vi "FPGA-MAIN.vi"() -> ()   [LabVIEW 2013]
uses:
  <vilib>/LabVIEW Targets/FPGA/cRIO/shared/nicrio_ModuleControls/nicrio_BasicConversionTime.ctl
  <vilib>/LabVIEW Targets/FPGA/cRIO/shared/nicrio_ModuleControls/nicrio_cRIO-9205_VoltageRange.ctl
  <vilib>/LabVIEW Targets/FPGA/cRIO/shared/nicrio_ModuleControls/nicrio_cRIO-9205_TerminalMode.ctl
  <vilib>/LabVIEW Targets/FPGA/cRIO/shared/nicrio_ModuleControls/nicrio_cRIO-9229_DataRatesRing.ctl
  <vilib>/rvi/Emulation/niFpgaSctlEmulationGetInTimedLoop.vi
  <vilib>/rvi/Emulation/niFpgaEmulationReportErrorSimple.vi
  <vilib>/rvi/Emulation/niFpgaGetClockAttributes.vi
  <vilib>/rvi/eio/common/nirviEmuTemplatePropertySet_errors.vi
  <vilib>/rvi/eio/common/nirviEmuTemplateMethod_errors.vi
  <vilib>/rvi/interface/RandomDataEmulation/nirviRandomDataFPGAFIFO.vi
  <vilib>/rvi/interface/RandomDataEmulation/niFpgaRandomDataHandleErrors.vi
  <vilib>/rvi/Emulation/niFpgaCriticalErrorInLSC.vi
  <vilib>/eio/EIOPropertyNode/EIOPropertyNode.xnode
  <vilib>/eio/EIONode/EIONode.xnode
  <vilib>/rvi/DataTransferAndStorage/Container/XNode/niFpgaContainer.xnode
  <vilib>/rvi/interface/RandomDataEmulation/nirviRandomDataFpgaReadWriteTemplate.vi
  <vilib>/eio/EIOMethodNode/EIOMethodNode.xnode
  <vilib>/rvi/eio/common/nirviEmuTemplatePropertyGet_errors.vi
  <vilib>/rvi/eio/common/nirviEmuTemplatePropertyGet_noerrors.vi
  <vilib>/rvi/eio/common/nirviEmuTemplatePropertySet_noerrors.vi
panel:
  in  "9229采样率":T1=1 items=["", "50.000 kS/s (NI 9229)", "25.000 kS/s (NI 9229)", "16.667 kS/s (NI 9229)", "12.500 kS/s (NI 9229)", "10.000 kS/s (NI 9229)", "8.333 kS/s (NI 9229)", "7.143 kS/s (NI 9229)", "6.250 kS/s (NI 9229)", "5.556 kS/s (NI 9229)", "5.000 kS/s (NI 9229)", "4.545 kS/s (NI 9229)", "4.167 kS/s (NI 9229)", "3.846 kS/s (NI 9229)", "3.571 kS/s (NI 9229)", "3.333 kS/s (NI 9229)", "3.125 kS/s (NI 9229)", "2.941 kS/s (NI 9229)", "2.778 kS/s (NI 9229)", "2.632 kS/s (NI 9229)", "2.500 kS/s (NI 9229)", "2.381 kS/s (NI 9229)", "2.273 kS/s (NI 9229)", "2.174 kS/s (NI 9229)", "2.083 kS/s (NI 9229)", "2.000 kS/s (NI 9229)", "1.923 kS/s (NI 9229)", "1.852 kS/s (NI 9229)", "1.786 kS/s (NI 9229)", "1.724 kS/s (NI 9229)", "1.667 kS/s (NI 9229)", "1.613 kS/s (NI 9229)"]
  out "9205循环值":u32=272
  out "9205/DI0":bool=TRUE
  out "9205fifo flower":bool
  in  "9205/DO0":bool
  out "9205fifo over":bool=TRUE
  out "9205fifo超时":bool=TRUE
  in  "9205Update AI Setings":bool
  in  "9205AI DEFINE":cluster{"AI通道":u8, "电压范围":T2, "接线端模式":T3}[](array[cluster])=[{"AI通道"=0, "电压范围"=enum."+/- 10V", "接线端模式"=enum."RSE"}, {"AI通道"=0, "电压范围"=enum."+/- 10V", "接线端模式"=enum."RSE"}, {"AI通道"=0, "电压范围"=enum."+/- 10V", "接线端模式"=enum."RSE"}, {"AI通道"=0, "电压范围"=enum."+/- 10V", "接线端模式"=enum."RSE"}, {"AI通道"=0, "电压范围"=enum."+/- 10V", "接线端模式"=enum."RSE"}, {"AI通道"=0, "电压范围"=enum."+/- 10V", "接线端模式"=enum."RSE"}, {"AI通道"=0, "电压范围"=enum."+/- 10V", "接线端模式"=enum."RSE"}, {"AI通道"=0, "电压范围"=enum."+/- 10V", "接线端模式"=enum."RSE"}, {"AI通道"=0, "电压范围"=enum."+/- 10V", "接线端模式"=enum."RSE"}, {"AI通道"=0, "电压范围"=enum."+/- 10V", "接线端模式"=enum."RSE"}, {"AI通道"=0, "电压范围"=enum."+/- 10V", "接线端模式"=enum."RSE"}, {"AI通道"=0, "电压范围"=enum."+/- 10V", "接线端模式"=enum."RSE"}, {"AI通道"=0, "电压范围"=enum."+/- 10V", "接线端模式"=enum."RSE"}, {"AI通道"=0, "电压范围"=enum."+/- 10V", "接线端模式"=enum."RSE"}, {"AI通道"=0, "电压范围"=enum."+/- 10V", "接线端模式"=enum."RSE"}, {"AI通道"=0, "电压范围"=enum."+/- 10V", "接线端模式"=enum."RSE"}, {"AI通道"=0, "电压范围"=enum."+/- 10V", "接线端模式"=enum."RSE"}, {"AI通道"=0, "电压范围"=enum."+/- 10V", "接线端模式"=enum."RSE"}, {"AI通道"=0, "电压范围"=enum."+/- 10V", "接线端模式"=enum."RSE"}, {"AI通道"=0, "电压范围"=enum."+/- 10V", "接线端模式"=enum."RSE"}, {"AI通道"=0, "电压范围"=enum."+/- 10V", "接线端模式"=enum."RSE"}, {"AI通道"=0, "电压范围"=enum."+/- 10V", "接线端模式"=enum."RSE"}, {"AI通道"=0, "电压范围"=enum."+/- 10V", "接线端模式"=enum."RSE"}, {"AI通道"=0, "电压范围"=enum."+/- 10V", "接线端模式"=enum."RSE"}, {"AI通道"=0, "电压范围"=enum."+/- 10V", "接线端模式"=enum."RSE"}]
  in  "9205Count(uSec)":u32 caption="计数器(uSec)"
  out "9213输出数据":T4
  out "9213通道状态":cluster{"超出范围":bool[], bool[]}
  in  "9213转换时间":T5
  in  "update9213":bool
  out "9229buff underflower":bool
  out "9229buff overflower":bool=TRUE
  in  "9229停止":bool
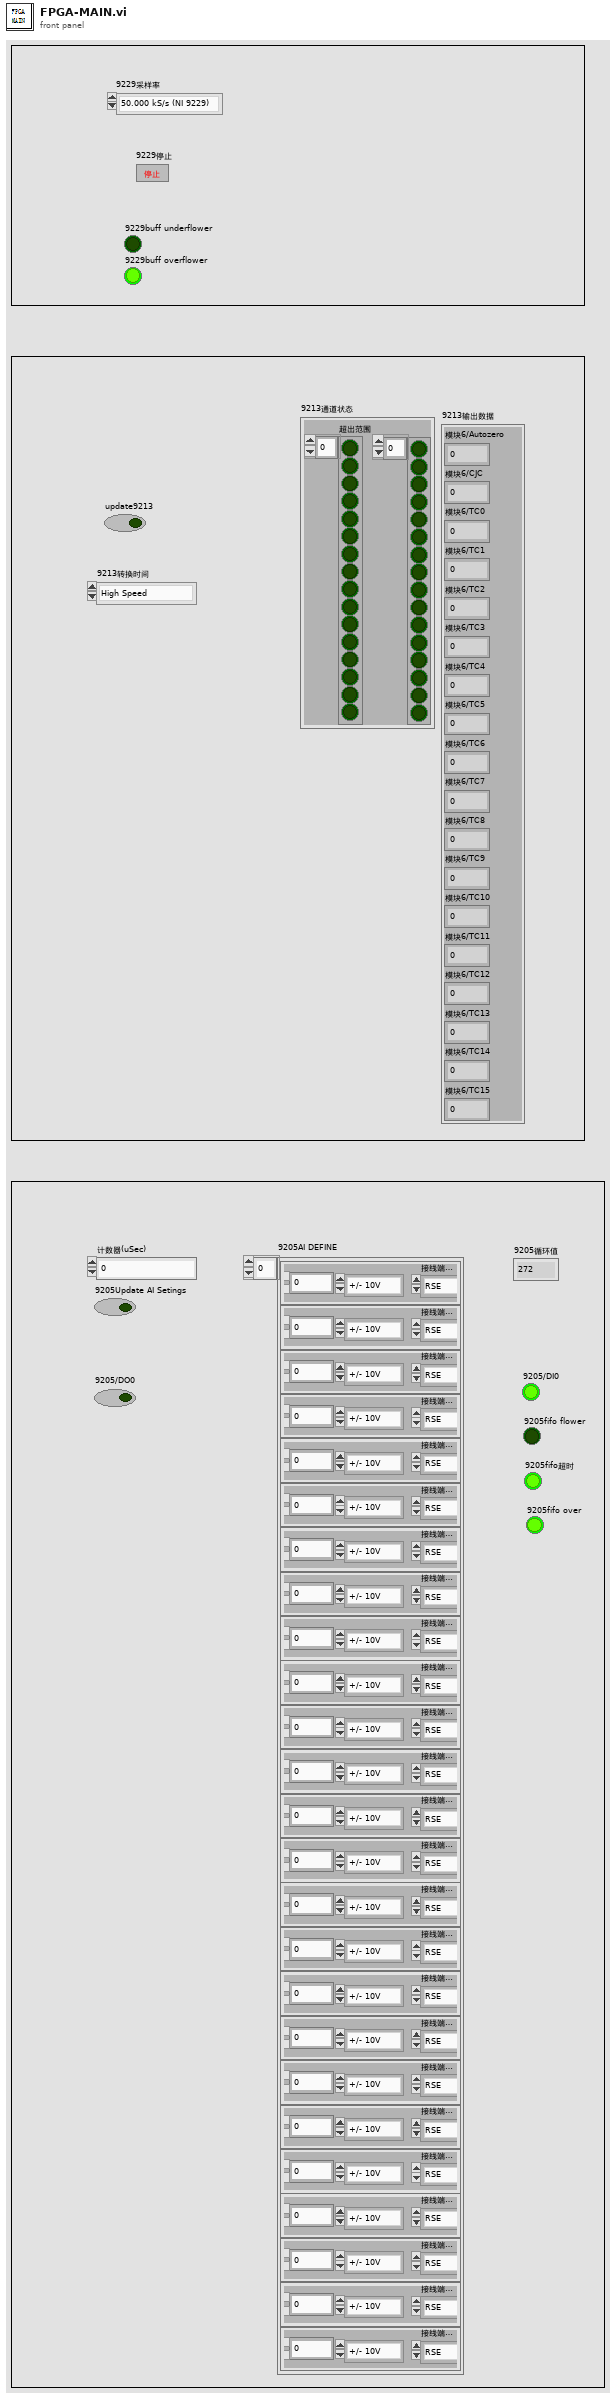
[diagram p1: front panel]
types:
  T1 = typedef "nicrio_cRIO-9229_DataRatesRing.ctl" = u8
  T2 = typedef "nicrio_cRIO-9205_VoltageRange.ctl" = enum8{"+/- 10V", "+/- 5V", "+/- 1V", "+/- 200mV"}
  T3 = typedef "nicrio_cRIO-9205_TerminalMode.ctl" = enum8{"RSE", "NRSE", "DIFF"}
  T4 = cluster{"模块6/Autozero":fxp<+/-,24,-2>, "模块6/CJC":fxp<+/-,24,-2>, "模块6/TC0":fxp<+/-,24,-2>, "模块6/TC1":fxp<+/-,24,-2>, "模块6/TC2":fxp<+/-,24,-2>, "模块6/TC3":fxp<+/-,24,-2>, "模块6/TC4":fxp<+/-,24,-2>, "模块6/TC5":fxp<+/-,24,-2>, "模块6/TC6":fxp<+/-,24,-2>, "模块6/TC7":fxp<+/-,24,-2>, "模块6/TC8":fxp<+/-,24,-2>, "模块6/TC9":fxp<+/-,24,-2>, "模块6/TC10":fxp<+/-,24,-2>, "模块6/TC11":fxp<+/-,24,-2>, "模块6/TC12":fxp<+/-,24,-2>, "模块6/TC13":fxp<+/-,24,-2>, "模块6/TC14":fxp<+/-,24,-2>, "模块6/TC15":fxp<+/-,24,-2>}
  T5 = typedef "nicrio_BasicConversionTime.ctl" = enum8{"High Speed", "High Resolution"}
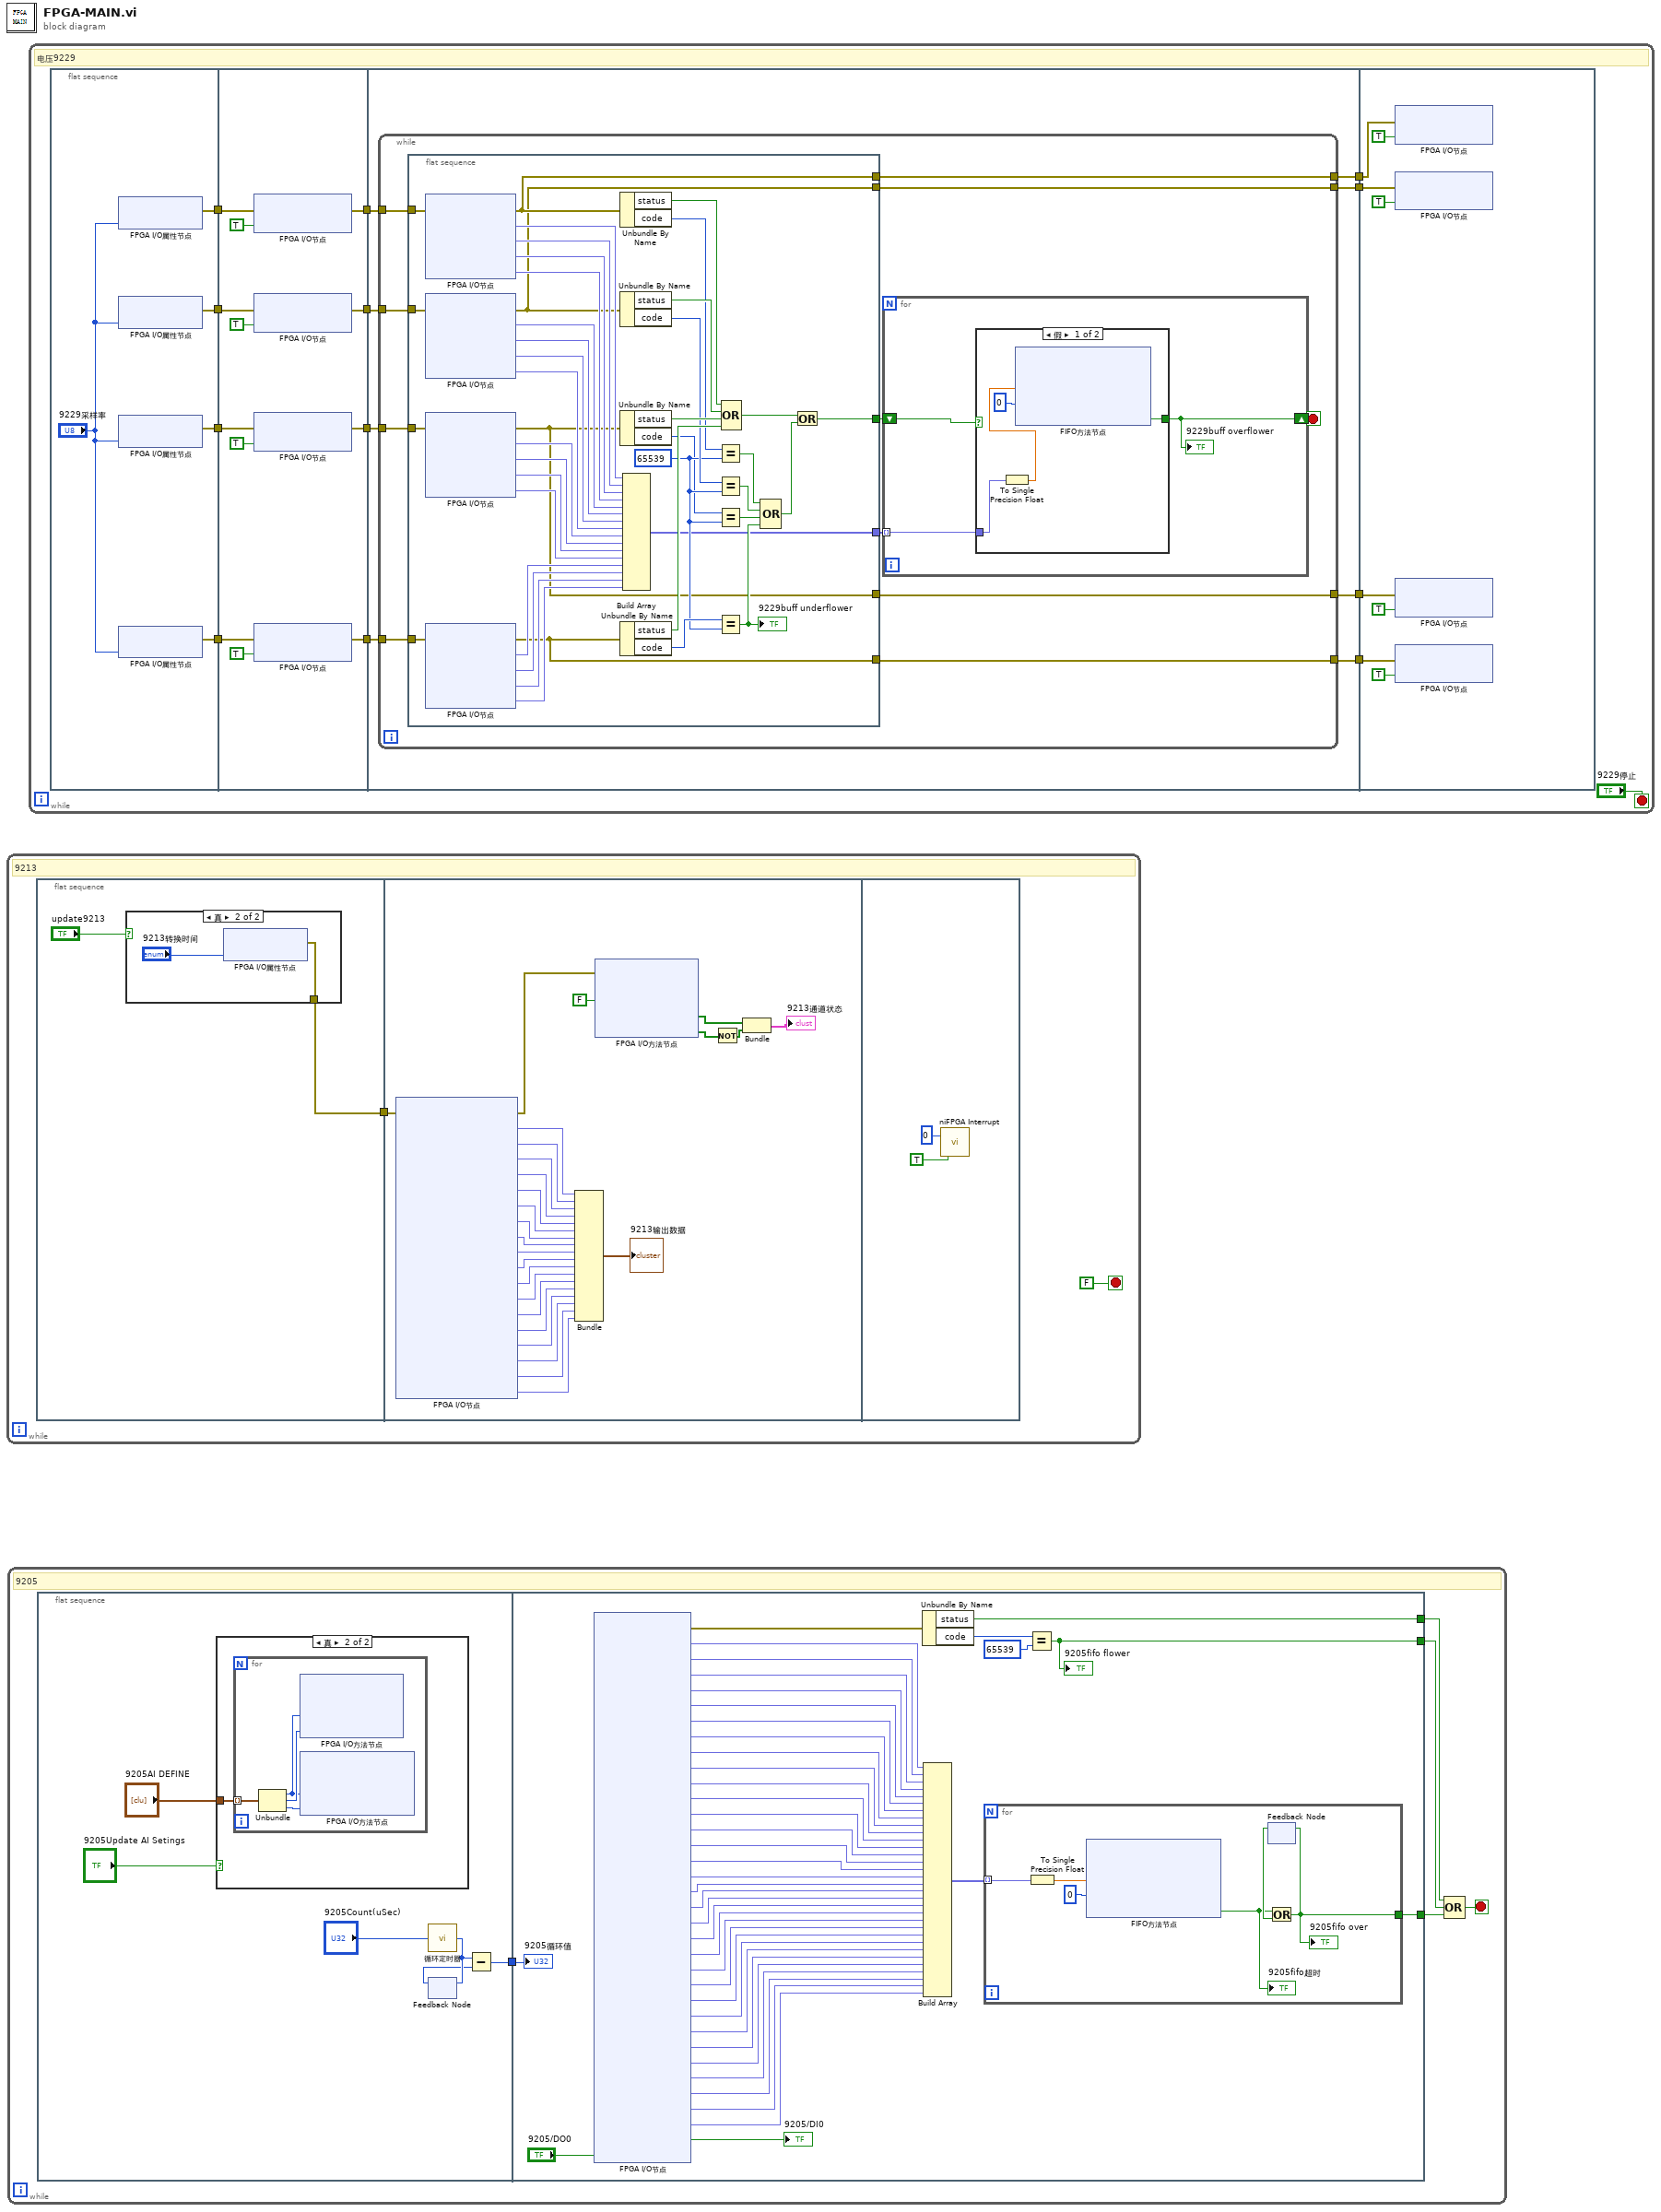
[diagram p0: block diagram]
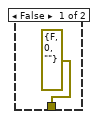
[diagram p3: hidden frame]
diagram:
  n1 = while {
    stop <- FALSE stop-if-true
    # "9213"
    n2 = flat-sequence {
      tunnel: [w3] -> w1
      tunnel: w1 -> [w14]
      frame #0 {
        n3 = case shown="真" "update9213" {
          tunnel: [errorcluster {"status"=FALSE, "code"=0, "source"=""} ("error out") w6] -> w3
          frame False {
          }
          frame True {
            n4 = xnode "FPGA I/O属性节点"("转换时间"="9213转换时间") -> ("error out"=w6:errorcluster)  [unwired: 2 in, 1 out]
          }
        }
      }
      frame #1 {
        n5 = xnode "FPGA I/O节点"("错误输入"=w14) -> ("错误输出"=w13:errorcluster, "模块6/Autozero"=w16:fxp<+/-,24,-2>, "模块6/CJC"=w17:fxp<+/-,24,-2>, "模块6/TC0"=w18:fxp<+/-,24,-2>, "模块6/TC1"=w19:fxp<+/-,24,-2>, "模块6/TC2"=w20:fxp<+/-,24,-2>, "模块6/TC3"=w21:fxp<+/-,24,-2>, "模块6/TC4"=w22:fxp<+/-,24,-2>, "模块6/TC5"=w23:fxp<+/-,24,-2>, "模块6/TC6"=w24:fxp<+/-,24,-2>, "模块6/TC7"=w25:fxp<+/-,24,-2>, "模块6/TC8"=w26:fxp<+/-,24,-2>, "模块6/TC9"=w27:fxp<+/-,24,-2>, "模块6/TC10"=w28:fxp<+/-,24,-2>, "模块6/TC11"=w29:fxp<+/-,24,-2>, "模块6/TC12"=w30:fxp<+/-,24,-2>, "模块6/TC13"=w31:fxp<+/-,24,-2>, "模块6/TC14"=w32:fxp<+/-,24,-2>, "模块6/TC15"=w33:fxp<+/-,24,-2>)  [unwired: 18 in, 18 out]
        n6 = Bundle("模块6/Autozero"=w16, "模块6/CJC"=w17, "模块6/TC0"=w18, "模块6/TC1"=w19, "模块6/TC2"=w20, "模块6/TC3"=w21, "模块6/TC4"=w22, "模块6/TC5"=w23, "模块6/TC6"=w24, "模块6/TC7"=w25, "模块6/TC8"=w26, "模块6/TC9"=w27, "模块6/TC10"=w28, "模块6/TC11"=w29, "模块6/TC12"=w30, "模块6/TC13"=w31, "模块6/TC14"=w32, "模块6/TC15"=w33) -> (→"9213输出数据":T4)  [unwired: 1 in]
        n7 = xnode "FPGA I/O方法节点"("error in"=w13, "强制状态读取"=FALSE) -> ("超出范围"=w10:bool[], "打开"=w11:bool[])  [unwired: 1 in, 2 out]
        n8 = Not(x=w11) -> (.not. x?=w9:bool[])
        n9 = Bundle("超出范围"=w10, w9) -> (→"9213通道状态":cluster{"超出范围":bool[], bool[]})  [unwired: 1 in]
      }
      frame #2 {
        n10 = call <vilib>:"niFPGA Interrupt.vi"("Wait Until Cleared (F)"=TRUE, "IRQ Number (0)"=u8 0) -> ()  [unwired: 1 in]
      }
    }
  }
  n11 = while {
    stop <- w40 stop-if-true
    # "9205"
    n12 = flat-sequence {
      tunnel: [w46] -> w39
      tunnel: w39 -> [w93]
      tunnel: [w55] -> w38
      tunnel: [w54] -> w37
      tunnel: [w53] -> w36
      frame #0 {
        n13 = case shown="真" "9205Update AI Setings" {
          tunnel: "9205AI DEFINE" -> [_ w47]
          frame False {
          }
          frame True {
            n14 = for {
              tunnel: w47 -> [w51] mode=indexing
              n15 = Unbundle(w51) -> ("AI通道"=w48:u8, "电压范围"=w50:T2, "接线端模式"=w49:T3)
              n16 = xnode "FPGA I/O方法节点"("AI通道"=w48, "电压范围"=w50) -> ()  [unwired: 1 in, 1 out]
              n17 = xnode "FPGA I/O方法节点"("AI通道"=w48, "接线端模式"=w49) -> ()  [unwired: 2 in, 2 out]
            }
          }
        }
        n18 = call "循环定时器"("Count(uSec)"="9205Count(uSec)") -> ("Tick Count(uSec)"=w43:u32)
        n19 = feedback #1() -> (w42:u32)  [unwired: 1 in]
        n20 = feedback-in #1(w43) -> ()
        n21 = Subtract(x=w43, y=w42) -> (x-y=w46:u32)
      }
      frame #1 {
        n22 = xnode "FPGA I/O节点"("模块7/DO0"="9205/DO0") -> ("错误输出"=w89:errorcluster, "模块7/AI0"=w56:fxp<+/-,26,5>, "模块7/AI1"=w57:fxp<+/-,26,5>, "模块7/AI2"=w58:fxp<+/-,26,5>, "模块7/AI3"=w59:fxp<+/-,26,5>, "模块7/AI4"=w60:fxp<+/-,26,5>, "模块7/AI5"=w61:fxp<+/-,26,5>, "模块7/AI6"=w62:fxp<+/-,26,5>, "模块7/AI7"=w63:fxp<+/-,26,5>, "模块7/AI8"=w64:fxp<+/-,26,5>, "模块7/AI9"=w65:fxp<+/-,26,5>, "模块7/AI10"=w66:fxp<+/-,26,5>, "模块7/AI11"=w67:fxp<+/-,26,5>, "模块7/AI12"=w68:fxp<+/-,26,5>, "模块7/AI13"=w69:fxp<+/-,26,5>, "模块7/AI14"=w70:fxp<+/-,26,5>, "模块7/AI15"=w71:fxp<+/-,26,5>, "模块7/AI16"=w72:fxp<+/-,26,5>, "模块7/AI17"=w73:fxp<+/-,26,5>, "模块7/AI18"=w74:fxp<+/-,26,5>, "模块7/AI19"=w75:fxp<+/-,26,5>, "模块7/AI20"=w76:fxp<+/-,26,5>, "模块7/AI21"=w77:fxp<+/-,26,5>, "模块7/AI22"=w78:fxp<+/-,26,5>, "模块7/AI23"=w79:fxp<+/-,26,5>, "模块7/AI24"=w80:fxp<+/-,26,5>, "模块7/AI25"=w81:fxp<+/-,26,5>, "模块7/AI26"=w82:fxp<+/-,26,5>, "模块7/AI27"=w83:fxp<+/-,26,5>, "模块7/AI28"=w84:fxp<+/-,26,5>, "模块7/AI29"=w85:fxp<+/-,26,5>, "模块7/AI30"=w86:fxp<+/-,26,5>, "模块7/AI31"=w87:fxp<+/-,26,5>, "模块7/DI0"=→"9205/DI0":bool)  [unwired: 35 in, 34 out]
        n23 = Unbundle By Name(w89) -> ("status"=w55:bool, "code"=w90:i32)
        n24 = Build Array(w56, w57, w58, w59, w60, w61, w62, w63, w64, w65, w66, w67, w68, w69, w70, w71, w72, w73, w74, w75, w76, w77, w78, w79, w80, w81, w82, w83, w84, w85, w86, w87) -> (w52:fxp<+/-,26,5>[])
        n25 = for {
          tunnel: [w95] -> w53
          tunnel: w52 -> [w94] mode=indexing
          n26 = To Single Precision Float(number=w94) -> (single precision float=w96:sgl)
          n27 = xnode ("FIFO方法节点")("元素"=w96, "超时"=0) -> ("超时？"=w97:bool)  [unwired: 1 in, 1 out]
          "9205fifo超时" <- w97
          n28 = feedback #2() -> (w98:bool)  [unwired: 1 in]
          n29 = Or(x=w97, y=w98) -> (x .or. y?=w95:bool)
          "9205fifo over" <- w95
          n30 = feedback-in #2(w95) -> ()
        }
        n31 = Equal?(x=w90, y=65539) -> (x = y?=w54:bool)
        "9205fifo flower" <- w54
        "9205循环值" <- w93
      }
    }
    n32 = Compound Arithmetic op=OR(w38, w37, w36) -> (w40:bool)
  }
  n33 = while {
    stop <- "9229停止" stop-if-true
    # "电压9229"
    n34 = flat-sequence {
      tunnel: [w117] -> w112
      tunnel: [w116] -> w111
      tunnel: [w115] -> w110
      tunnel: [w114] -> w109
      tunnel: w112 -> [w125]
      tunnel: w111 -> [w124]
      tunnel: w110 -> [w123]
      tunnel: w109 -> [w122]
      tunnel: [w121] -> w108
      tunnel: [w120] -> w107
      tunnel: [w119] -> w106
      tunnel: [w118] -> w105
      tunnel: w108 -> [w137]
      tunnel: w107 -> [w136]
      tunnel: w106 -> [w135]
      tunnel: w105 -> [w134]
      tunnel: [w133] -> w104
      tunnel: [w132] -> w103
      tunnel: [w131] -> w102
      tunnel: [w130] -> w101
      tunnel: w104 -> [w205]
      tunnel: w103 -> [w204]
      tunnel: w102 -> [w203]
      tunnel: w101 -> [w202]
      frame #0 {
        n35 = xnode "FPGA I/O属性节点"("采样率"="9229采样率") -> ("error out"=w117:errorcluster)  [unwired: 2 in, 1 out]
        n36 = xnode "FPGA I/O属性节点"("采样率"="9229采样率") -> ("error out"=w116:errorcluster)  [unwired: 2 in, 1 out]
        n37 = xnode "FPGA I/O属性节点"("采样率"="9229采样率") -> ("error out"=w115:errorcluster)  [unwired: 2 in, 1 out]
        n38 = xnode "FPGA I/O属性节点"("采样率"="9229采样率") -> ("error out"=w114:errorcluster)  [unwired: 2 in, 1 out]
      }
      frame #1 {
        n39 = xnode "FPGA I/O节点"("错误输入"=w125, "模块2/Start"=TRUE) -> ("错误输出"=w121:errorcluster)  [unwired: 1 in, 1 out]
        n40 = xnode "FPGA I/O节点"("错误输入"=w124, "模块3/Start"=TRUE) -> ("错误输出"=w120:errorcluster)  [unwired: 1 in, 1 out]
        n41 = xnode "FPGA I/O节点"("错误输入"=w123, "模块4/Start"=TRUE) -> ("错误输出"=w119:errorcluster)  [unwired: 1 in, 1 out]
        n42 = xnode "FPGA I/O节点"("错误输入"=w122, "模块5/Start"=TRUE) -> ("错误输出"=w118:errorcluster)  [unwired: 1 in, 1 out]
      }
      frame #2 {
        n43 = while {
          tunnel: w137 -> [w148]
          tunnel: w136 -> [w147]
          tunnel: w135 -> [w146]
          tunnel: w134 -> [w145]
          tunnel: [w142] -> w133
          tunnel: [w141] -> w132
          tunnel: [w140] -> w131
          tunnel: [w139] -> w130
          stop <- w138 stop-if-true
          n44 = flat-sequence {
            tunnel: w148 -> [w197]
            tunnel: w147 -> [w196]
            tunnel: w146 -> [w195]
            tunnel: w145 -> [w194]
            tunnel: [w162] -> w144
            tunnel: [w161] -> w143
            tunnel: [w160] -> w142
            tunnel: [w159] -> w141
            tunnel: [w158] -> w140
            tunnel: [w157] -> w139
            frame #0 {
              w170 = 65539
              n45 = xnode "FPGA I/O节点"("错误输入"=w197) -> ("错误输出"=w160:errorcluster, "模块2/AI0"=w193:fxp<+/-,24,7>, "模块2/AI1"=w192:fxp<+/-,24,7>, "模块2/AI2"=w191:fxp<+/-,24,7>, "模块2/AI3"=w190:fxp<+/-,24,7>)  [unwired: 4 in, 4 out]
              n46 = xnode "FPGA I/O节点"("错误输入"=w196) -> ("错误输出"=w159:errorcluster, "模块3/AI0"=w189:fxp<+/-,24,7>, "模块3/AI1"=w188:fxp<+/-,24,7>, "模块3/AI2"=w187:fxp<+/-,24,7>, "模块3/AI3"=w186:fxp<+/-,24,7>)  [unwired: 4 in, 4 out]
              n47 = xnode "FPGA I/O节点"("错误输入"=w195) -> ("错误输出"=w158:errorcluster, "模块4/AI0"=w185:fxp<+/-,24,7>, "模块4/AI1"=w184:fxp<+/-,24,7>, "模块4/AI2"=w183:fxp<+/-,24,7>, "模块4/AI3"=w182:fxp<+/-,24,7>)  [unwired: 4 in, 4 out]
              n48 = xnode "FPGA I/O节点"("错误输入"=w194) -> ("错误输出"=w157:errorcluster, "模块5/AI0"=w181:fxp<+/-,24,7>, "模块5/AI1"=w180:fxp<+/-,24,7>, "模块5/AI2"=w179:fxp<+/-,24,7>, "模块5/AI3"=w178:fxp<+/-,24,7>)  [unwired: 4 in, 4 out]
              n49 = Unbundle By Name(w160) -> ("status"=w177:bool, "code"=w172:i32)
              n50 = Unbundle By Name(w159) -> ("status"=w176:bool, "code"=w171:i32)
              n51 = Unbundle By Name(w158) -> ("status"=w175:bool, "code"=w169:i32)
              n52 = Unbundle By Name(w157) -> ("status"=w174:bool, "code"=w173:i32)
              n53 = Build Array(w193, w192, w191, w190, w189, w188, w187, w186, w185, w184, w183, w182, w181, w180, w179, w178) -> (w161:fxp<+/-,24,7>[])
              n54 = Equal?(x=w172, y=w170) -> (x = y?=w168:bool)
              n55 = Equal?(x=w171, y=w170) -> (x = y?=w167:bool)
              n56 = Equal?(x=w169, y=w170) -> (x = y?=w166:bool)
              n57 = Equal?(x=w173, y=w170) -> (x = y?=w165:bool)
              "9229buff underflower" <- w165
              n58 = Compound Arithmetic op=OR(w177, w176, w175, w174) -> (w164:bool)
              n59 = Compound Arithmetic op=OR(w168, w167, w166, w165) -> (w163:bool)
              n60 = Or(x=w164, y=w163) -> (x .or. y?=w162:bool)
            }
          }
          n61 = for {
            shift-right: [w151] -> w138
            shift-left: w144 -> [w149]
            tunnel: w143 -> [w150] mode=indexing
            n62 = case shown="假" w149 {
              selector: w149 -> [_ w156]
              tunnel: [w154 w156] -> w151
              tunnel: w150 -> [w153 _]
              frame False {
                n63 = To Single Precision Float(number=w153) -> (single precision float=w152:sgl)
                n64 = xnode ("FIFO方法节点")("元素"=w152, "超时"=0) -> ("超时？"=w154:bool)  [unwired: 1 in, 1 out]
              }
              frame True {
              }
            }
            "9229buff overflower" <- w151
          }
        }
      }
      frame #3 {
        n65 = xnode "FPGA I/O节点"("错误输入"=w205, "模块2/Stop"=TRUE) -> ()  [unwired: 1 in, 2 out]
        n66 = xnode "FPGA I/O节点"("错误输入"=w204, "模块3/Stop"=TRUE) -> ()  [unwired: 1 in, 2 out]
        n67 = xnode "FPGA I/O节点"("错误输入"=w203, "模块4/Stop"=TRUE) -> ()  [unwired: 1 in, 2 out]
        n68 = xnode "FPGA I/O节点"("错误输入"=w202, "模块5/Stop"=TRUE) -> ()  [unwired: 1 in, 2 out]
      }
    }
  }
